vi "_RT_Pub_RT_Restart.vi"(8 "error in (no error)":errorcluster, 10 "Safe Mode?":bool) -> (0 "error out":errorcluster)   [LabVIEW 2018]
uses:
  <vilib>/nisyscfg/Close (System).vi
  <vilib>/nisyscfg/nisyscfg.lvlib
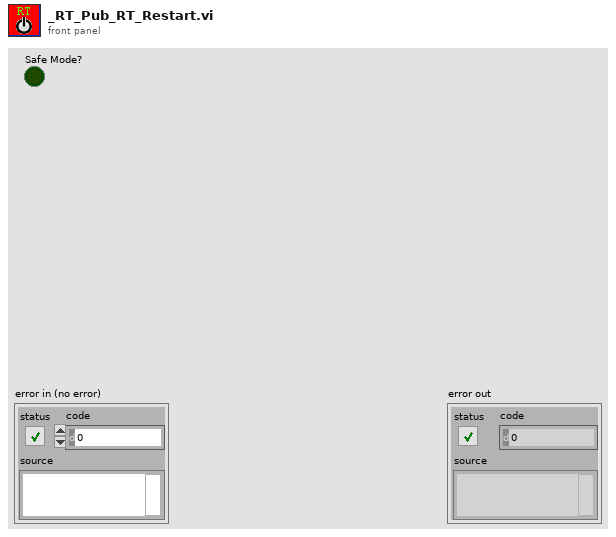
[diagram p1: front panel]
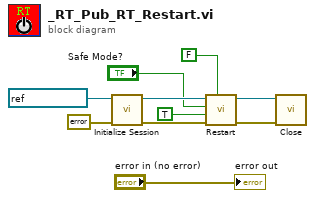
[diagram p0: block diagram]
diagram:
  n1 = call <vilib>:"Initialize Session.vi"("error in (no error)"=errorcluster {"status"=FALSE, "code"=0, "source"=""}, "Target (localhost)"=refnum<k21> "localhost") -> ("error out"=w7:errorcluster, "Session out"=w10:refnum<k21>)  [unwired: 8 in]
  n2 = call <vilib>:"Restart.vi"("Wait Until Complete (T)"=FALSE, "error in (no error)"=w7, "Flush DNS (F)"=TRUE, "Install Mode (F)"="Safe Mode?", "Session in"=w10) -> ("error out"=w9:errorcluster, "Session out"=w8:refnum<k21>)  [unwired: 4 in, 1 out]
  n3 = call-poly <vilib>:"Close.vi"("error in (no error)"=w9, "Session in"=w8) -> ()  [unwired: 9 in, 1 out]
  "error out" <- "error in (no error)"
